vi "writetofile.vi"(6 "FilePath":refnum<vi>, 7 "Save Flag Reference":refnum<vi>, 8 "error in (no error)":errorcluster, 9 "Rec Flag Reference":refnum<vi>, 10 "Stop Flag Reference":refnum<vi>, 11 "Imaging in":refnum<class "Imaging.lvclass">) -> (0 "error out":errorcluster, 3 "Imaging out":refnum<class "Imaging.lvclass">)   [LabVIEW 2014, in "Imaging.lvclass"]
uses:
  Imaging.lvclass
  Imaging.lvclass/Imaging.ctl
  private/HDF5Tools32/LabView/Append To Dataset 2D Double.vi
  private/HDF5Tools32/LabView/HDF5Tools.lvlib
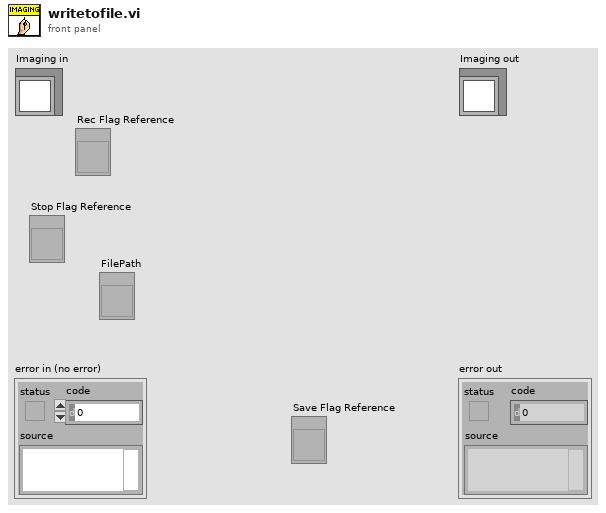
[diagram p1: front panel]
types:
  T1 = typedef "AviRefnum.ctl" = refnum<k1>
  T2 = typedef "IMAQ Image.ctl" = refnum<image>
  T3 = cluster{"Image Out":T2, dbl, "seconds since 1Jan1904":timestamp}
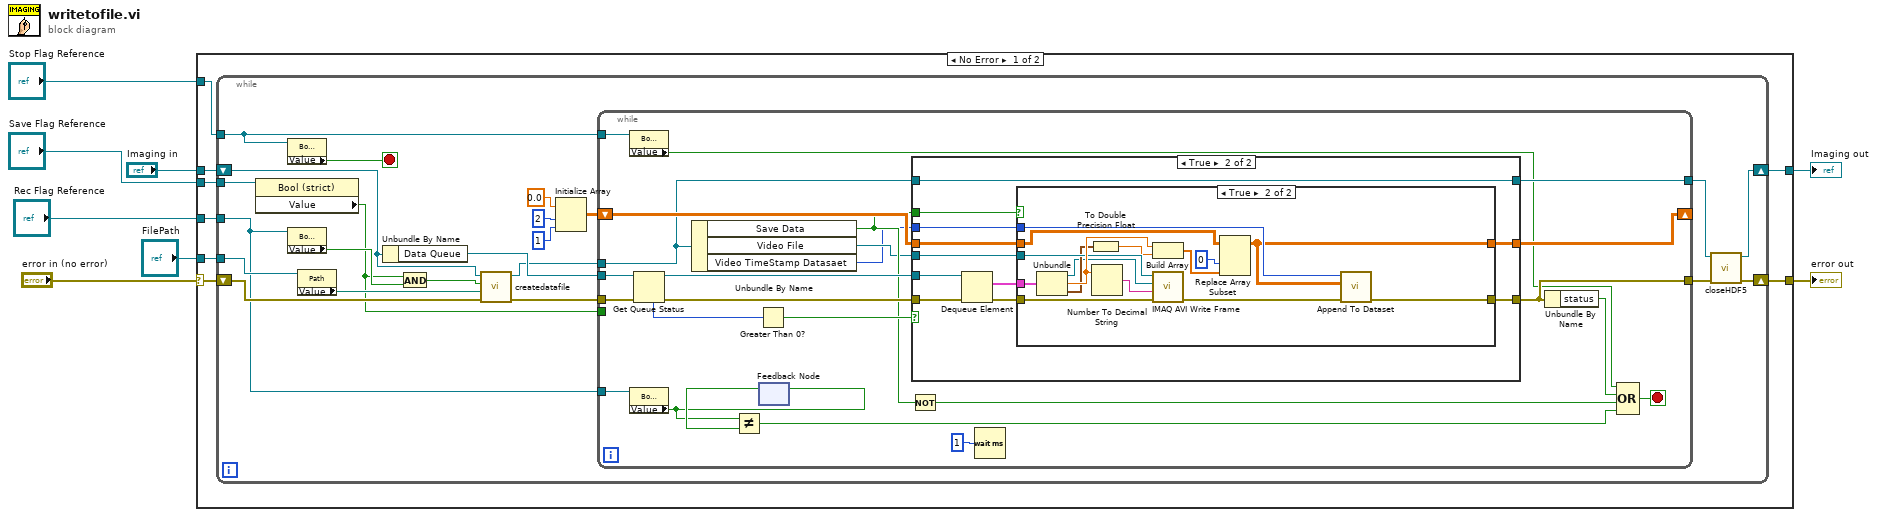
[diagram p0: block diagram]
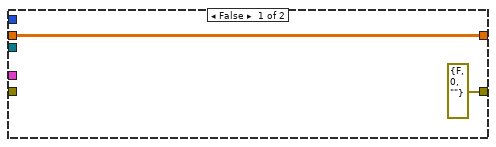
[diagram p3: hidden frame]
diagram:
  n1 = case shown="No Error" "error in (no error)" {
    selector: "error in (no error)" -> [w14 w95]
    tunnel: [w12 w95] -> w7
    tunnel: "Imaging in" -> [w15 w94]
    tunnel: "Stop Flag Reference" -> [w16 _]
    tunnel: [w13 w94] -> w4
    tunnel: "Rec Flag Reference" -> [w11 _]
    tunnel: "FilePath" -> [w10 _]
    tunnel: "Save Flag Reference" -> [w9 _]
    frame No Error {
      n2 = while {
        tunnel: w16 -> [w25]
        shift-right: [w27] -> w13
        shift-left: w15 -> [w33]
        shift-right: [w26] -> w12
        shift-left: w14 -> [w31]
        tunnel: w11 -> [w19]
        tunnel: w10 -> [w24]
        tunnel: w9 -> [w17]
        stop <- w20 stop-if-true
        n3 = property class="Bool (strict)"(reference=w17) -> ("Value"=w18:bool)  [unwired: 1 in, 2 out]
        n4 = property class="Bool (strict)"(reference=w25) -> ("Value"=w20:bool)  [unwired: 1 in, 2 out]
        n5 = property class="Bool (strict)"(reference=w19) -> ("Value"=w22:bool)  [unwired: 1 in, 2 out]
        n6 = property class="Path"(reference=w24) -> ("Value"=w23:path)  [unwired: 1 in, 2 out]
        n7 = Unbundle By Name(w33) -> ("Data Queue"=w38:refnum<queue>)
        n8 = And(x=w18, y=w22) -> (x .and. y?=w21:bool)
        n9 = call-dynamic "createdatafile.vi"("error in (no error)"=w31, "File Path"=w23, "Save Video"=w21, "Imaging in"=w33) -> ("error out"=w30:errorcluster, "Imaging out"=w32:refnum<class "Imaging.lvclass">)  [unwired: 6 in]
        n10 = Initialize Array(0.0 ("element"), 2 ("dimension size"), 1 ("dimension size")) -> (w34:dbl[][])
        n11 = while {
          tunnel: w30 -> [w62]
          tunnel: [w59] -> w28
          tunnel: w25 -> [w60]
          tunnel: w38 -> [w58]
          tunnel: w32 -> [w43]
          tunnel: [w57] -> w29
          shift-right: [w51] -> _
          shift-left: w34 -> [w52]
          tunnel: w18 -> [_]
          tunnel: w19 -> [w42]
          stop <- w48 stop-if-true
          n12 = property class="Bool (strict)"(reference=w60) -> ("Value"=w50:bool)  [unwired: 1 in, 2 out]
          n13 = property class="Bool (strict)"(reference=w42) -> ("Value"=w40:bool)  [unwired: 1 in, 2 out]
          n14 = Get Queue Status(queue=w58, error in (no error)=w62) -> (queue out=w53:refnum<queue>, error out=w61:errorcluster, # elements in queue=w55:i32)  [unwired: 1 in, 5 out]
          n15 = Unbundle By Name(w43) -> ("Save Data"=w46:bool, "Video File"=w45:T1, "Video TimeStamp Datasaet"=w44:i32)
          n16 = Greater Than 0?(x=w55) -> (x > 0?=w56:bool)
          n17 = feedback-in #1(w40) -> ()
          n18 = feedback #1() -> (w41:bool)  [unwired: 1 in]
          n19 = Not Equal?(x=w40, y=w41) -> (x != y?=w39:bool)
          n20 = Not(x=w46) -> (.not. x?=w47:bool)
          n21 = case shown="True" w56 {
            tunnel: w61 -> [w65 w73]
            tunnel: [w65 w71] -> w59
            tunnel: w43 -> [w64 w74]
            tunnel: [w64 w74] -> w57
            tunnel: w53 -> [_ w76]
            tunnel: w52 -> [w63 w70]
            tunnel: [w63 w69] -> w51
            tunnel: w46 -> [_ w68]
            tunnel: w45 -> [_ w67]
            tunnel: w44 -> [_ w66]
            frame False {
            }
            frame True {
              n22 = Dequeue Element(queue=w76, error in (no error)=w73) -> (element=w75:T3, error out=w72:errorcluster)  [unwired: 1 in, 2 out]
              n23 = case shown="True" w68 {
                tunnel: [errorcluster {"status"=FALSE, "code"=0, "source"=""} ("Error out") w87] -> w71
                tunnel: w75 -> [_ w93]
                tunnel: w67 -> [_ w90]
                tunnel: w66 -> [_ w89]
                tunnel: w72 -> [_ w81]
                tunnel: w70 -> [w77 w84]
                tunnel: [w77 w82] -> w69
                frame False {
                }
                frame True {
                  n24 = Unbundle(w93) -> ("Image Out"=w80:T2, w91:dbl, "seconds since 1Jan1904"=w85:timestamp)
                  n25 = To Double Precision Float(number=w85) -> (double precision float=w86:dbl)
                  n26 = Number To Decimal String(number=w91) -> (decimal integer string=w92:string)  [unwired: 1 in]
                  n27 = Build Array(w91, w86) -> (w83:dbl[])
                  n28 = call "IMAQ AVI Write Frame"("error in (no error)"=w81, "Data"=w92, "Image"=w80, "Avi Refnum"=w90) -> ("error out"=w88:errorcluster)  [unwired: 7 out]
                  n29 = Replace Array Subset(array=w84, new element=w83, index (col)=0 ("disabled index (col)")) -> (w82:dbl[][])  [unwired: 1 in]
                  n30 = call-poly "Append To Dataset.vi"("Error in (no error)"=w88, "Data"=w82, "Dataset id in"=w89) -> ("Error out"=w87:errorcluster)  [unwired: 7 in, 1 out]
                }
              }
            }
          }
          n31 = Wait (ms)(milliseconds to wait=u32 1) -> ()  [unwired: 1 out]
          n32 = Unbundle By Name(w59) -> ("status"=w49:bool)
          n33 = Compound Arithmetic op=OR(w50, w49, w47, w39) -> (w48:bool)
        }
        n34 = call-dynamic "closeHDF5.vi"("error in (no error)"=w28, "Imaging in"=w29) -> ("error out"=w26:errorcluster, "Imaging out"=w27:refnum<class "Imaging.lvclass">)  [unwired: 8 in]
      }
    }
    frame Error {
    }
  }
  "error out" <- w7
  "Imaging out" <- w4
